vi "Read Photoresistor Array.vi"() -> (3 "0, 1":i16[](array[numeric]))   [LabVIEW 2018]
uses:
  <vilib>/myRIO/Instrument Drivers/Onboard IO/DIO/typedefs/DIO Reference.ctl
  <vilib>/myRIO/Common/Instrument Driver Framework/Utilities/typedefs/myRIO Generic Hardware Reference.ctl
  <vilib>/myRIO/Common/Instrument Driver Framework/Utilities/typedefs/Hardware Version Enum.ctl
  <vilib>/myRIO/Common/Instrument Driver Framework/Utilities/typedefs/myRIO v1.0 Reference.ctl
  <vilib>/myRIO/Common/Instrument Driver Framework/Utilities/typedefs/Generic FPGA Reference.ctl
  <vilib>/myRIO/Common/Instrument Driver Framework/myRIO v1.0/DIO/typedefs/DIO Channels List.ctl
  <vilib>/myRIO/Common/Instrument Driver Framework/myRIO v1.0/DIO/typedefs/DIO Channels Enum.ctl
  <vilib>/userdefined/High Color/nirio_resource_hc.ctl
  <vilib>/myRIO/Common/Instrument Driver Framework/Utilities/vis/Is FPGA Ref Available.vi
  <vilib>/myRIO/Common/Instrument Driver Framework/myRIO v1.0/DIO/vis/myRIO v1.1 Open DIO.vi
  <vilib>/myRIO/Instrument Drivers/Onboard IO/DIO/vis/Read.vi
  <vilib>/myRIO/Common/Instrument Driver Framework/Utilities/vis/Validate Channels.vi
  <vilib>/myRIO/Common/Instrument Driver Framework/myRIO v1.0/DIO/vis/myRIO v1.0 Reserve DIO.vi
  <vilib>/myRIO/Common/Instrument Driver Framework/myRIO v1.0/Resource Manager/vis/myRIO v1.0 Reserve Channel List.vi
  <vilib>/myRIO/Common/Instrument Driver Framework/myRIO v1.0/DIO/vis/myRIO v1.0 Build MUX Configuration DIO.vi
  <vilib>/myRIO/Common/Instrument Driver Framework/myRIO v1.0/Resource Manager/vis/myRIO v1.0 Reserve Channel.vi
  <vilib>/myRIO/Common/Instrument Driver Framework/myRIO v1.0/Resource Manager/vis/myRIO v1.0 Unreserve Channel.vi
  <vilib>/myRIO/Common/Instrument Driver Framework/myRIO v1.0/Resource Manager/vis/myRIO v1.0 Create Configuration List.vi
  <vilib>/myRIO/Common/Instrument Driver Framework/myRIO v1.0/Resource Manager/vis/myRIO v1.0 Build Mutex Name.vi
  <vilib>/Utility/VariantDataType/GetNumericInfo.vi
  <vilib>/Utility/error.llb/Error Cluster From Error Code.vi
  <vilib>/myRIO/Common/Instrument Driver Framework/myRIO v1.0/myRIO v1.1 Open.vi
  <vilib>/myRIO/Common/Instrument Driver Framework/Utilities/vis/IO Manager.vi
  <vilib>/myRIO/Common/Instrument Driver Framework/Utilities/vis/Configuration Manager.vi
  <vilib>/myRIO/Common/Instrument Driver Framework/myRIO v1.0/Resource Manager/vis/myRIO v1.0 Configure IO.vi
  <vilib>/myRIO/Common/Instrument Driver Framework/myRIO v1.0/myRIO v1.0 Close.vi
  <vilib>/myRIO/Common/Instrument Driver Framework/myRIO v1.0/DIO/vis/myRIO v1.0 Read DIO.vi
  <vilib>/myRIO/Express VI/Onboard IO/DI/DI Express VI.xnode
  <vilib>/myRIO/Instrument Drivers/Onboard IO/DIO/vis/myRIO DIO Open.xnode
  <vilib>/myRIO/Instrument Drivers/Onboard IO/DIO/DIO.lvlib
panel:
  out "size(s)":i32
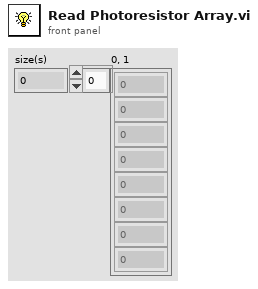
[diagram p1: front panel]
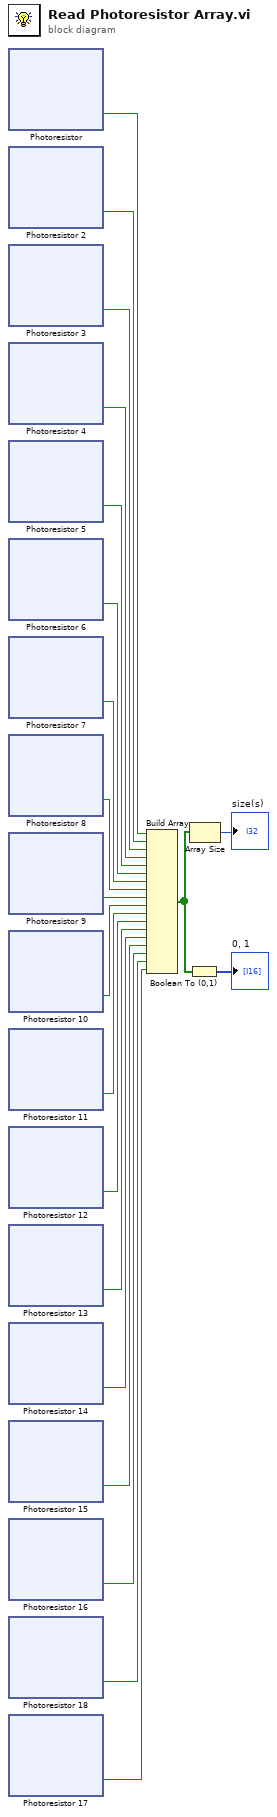
[diagram p0: block diagram]
diagram:
  n1 = xnode "Photoresistor"() -> ("A/DIO0 (Pin 11)"=w21:bool)  [unwired: 1 in, 1 out]
  n2 = xnode "Photoresistor 2"() -> ("A/DIO1 (Pin 13)"=w20:bool)  [unwired: 1 in, 1 out]
  n3 = xnode "Photoresistor 3"() -> ("A/DIO2 (Pin 15)"=w19:bool)  [unwired: 1 in, 1 out]
  n4 = xnode "Photoresistor 4"() -> ("A/DIO3 (Pin 17)"=w18:bool)  [unwired: 1 in, 1 out]
  n5 = xnode "Photoresistor 5"() -> ("A/DIO4 (Pin 19)"=w17:bool)  [unwired: 1 in, 1 out]
  n6 = xnode "Photoresistor 6"() -> ("A/DIO5 (Pin 21)"=w16:bool)  [unwired: 1 in, 1 out]
  n7 = xnode "Photoresistor 7"() -> ("A/DIO6 (Pin 23)"=w15:bool)  [unwired: 1 in, 1 out]
  n8 = xnode "Photoresistor 8"() -> ("A/DIO7 (Pin 25)"=w14:bool)  [unwired: 1 in, 1 out]
  n9 = xnode "Photoresistor 9"() -> ("A/DIO8 (Pin 27)"=w13:bool)  [unwired: 1 in, 1 out]
  n10 = xnode "Photoresistor 10"() -> ("A/DIO9 (Pin 29)"=w12:bool)  [unwired: 1 in, 1 out]
  n11 = xnode "Photoresistor 11"() -> ("A/DIO10 (Pin 31)"=w11:bool)  [unwired: 1 in, 1 out]
  n12 = xnode "Photoresistor 12"() -> ("A/DIO11 (Pin 18)"=w10:bool)  [unwired: 1 in, 1 out]
  n13 = xnode "Photoresistor 13"() -> ("A/DIO12 (Pin 22)"=w9:bool)  [unwired: 1 in, 1 out]
  n14 = xnode "Photoresistor 14"() -> ("A/DIO13 (Pin 26)"=w8:bool)  [unwired: 1 in, 1 out]
  n15 = xnode "Photoresistor 15"() -> ("A/DIO14 (Pin 32)"=w7:bool)  [unwired: 1 in, 1 out]
  n16 = xnode "Photoresistor 16"() -> ("A/DIO15 (Pin 34)"=w6:bool)  [unwired: 1 in, 1 out]
  n17 = xnode "Photoresistor 18"() -> ("B/DIO14 (Pin 32)"=w2:bool)  [unwired: 1 in, 1 out]
  n18 = xnode "Photoresistor 17"() -> ("B/DIO15 (Pin 34)"=w1:bool)  [unwired: 1 in, 1 out]
  n19 = Build Array(w21, w20, w19, w18, w17, w16, w15, w14, w13, w12, w11, w10, w9, w8, w7, w6, w2, w1) -> (w4:bool[])
  n20 = Boolean To (0,1)(Boolean=w4) -> (0, 1=→"0, 1":i16[])
  n21 = Array Size(array=w4) -> (size(s)=→"size(s)":i32)
